vi "LNLS Control LOCON_BIPOLAR_16BITS Data to PS Data.vi"(8 "error in (no error)":errorcluster, 11 "PS Setpoints LOCON Data":T1[](array[typedef]) {"status" format="%08b"}) -> (0 "error out":errorcluster, 2 "PS Status":bool[](array[boolean]), 3 "PS Setpoints":dbl[](array[numeric]))   [LabVIEW 2011, in "LNLS Control VIs.lvlib"]
uses:
  LNLS Control VIs.lvlib
  Types Definitions/Type LOCON_BIPOLAR_16BITS.ctl
  Type Definitions.lvlib
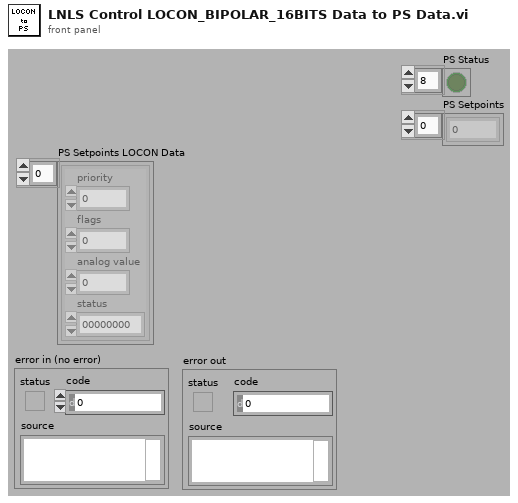
[diagram p1: front panel]
types:
  T1 = typedef "Type Definitions.lvlib/Type LOCON_BIPOLAR_16BITS.ctl" = cluster{"priority":u8, "flags":u8, "analog value":u16, "status":u8}
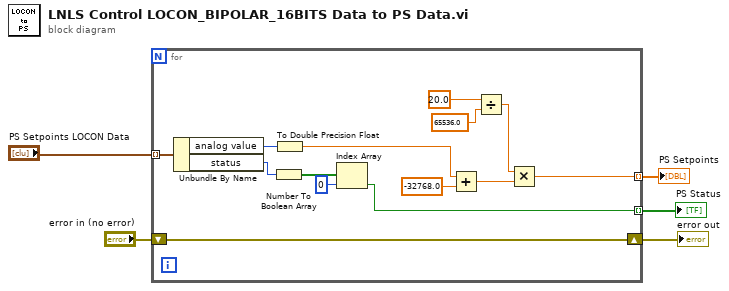
[diagram p0: block diagram]
diagram:
  n1 = for {
    tunnel: "PS Setpoints LOCON Data" -> [w19] mode=indexing
    shift-right: [w14] -> w3
    shift-left: "error in (no error)" -> [w14]
    tunnel: [w7] -> w1 mode=indexing
    tunnel: [w6] -> w2 mode=indexing
    n2 = Unbundle By Name(w19) -> ("analog value"=w18:u16, "status"=w17:u8)
    n3 = Number To Boolean Array(number=w17) -> (Boolean array=w16:bool[])
    n4 = To Double Precision Float(number=w18) -> (double precision float=w9:dbl)
    n5 = Index Array(array=w16, index=0) -> (element=w6:bool)
    n6 = Add(x=w9, y=-32768.0) -> (x+y=w8:dbl)
    n7 = Divide(x=20.0, y=65536.0) -> (x/y=w12:dbl)
    n8 = Multiply(x=w12, y=w8) -> (x*y=w7:dbl)
  }
  "error out" <- w3
  "PS Status" <- w2
  "PS Setpoints" <- w1
